vi "Create_Probe_Box.vi"(1 "Probe Volume":T1=[{"Max"=15.0, "Min"=-15.0}, {"Max"=250.0, "Min"=0.0}, {"Max"=15.0, "Min"=-15.0}] {"Min" format="%#.1f"; "Max" format="%#.1f"}, 2 "Probe Position":sgl[](array[numeric]) format="%.2f") -> (0 "Current Probe Volume":T1=[{"Max"=15.0, "Min"=-15.0}, {"Max"=250.0, "Min"=0.0}, {"Max"=15.0, "Min"=-15.0}] {"Min" format="%#.1f"; "Max" format="%#.1f"})   [LabVIEW 2014]
uses:
  Box_size.ctl
panel:
  # "(Relative to measurement position)"
  # "X                           Y                          Z"
  # "X                Y                  Z"
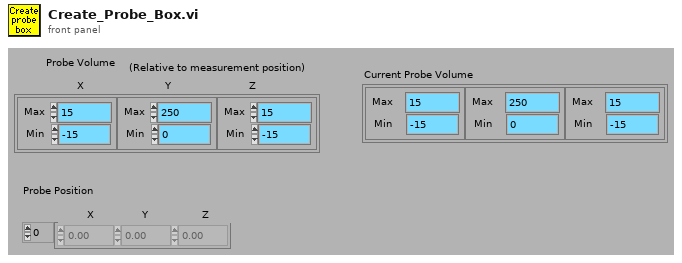
[diagram p1: front panel]
types:
  T1 = typedef "Box_size.ctl" = cluster{"Max":sgl, "Min":sgl}[]
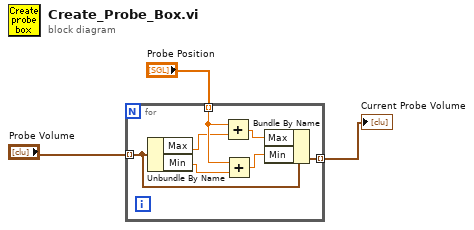
[diagram p0: block diagram]
diagram:
  n1 = for {
    tunnel: "Probe Volume" -> [w7] mode=indexing
    tunnel: "Probe Position" -> [w10] mode=indexing
    tunnel: [w4] -> w2 mode=indexing
    n2 = Unbundle By Name(w7) -> ("Max"=w9:sgl, "Min"=w8:sgl)
    n3 = Add(x=w10, y=w9) -> (x+y=w6:sgl)
    n4 = Add(x=w10, y=w8) -> (x+y=w5:sgl)
    n5 = Bundle By Name(cluster=w7, "Max"=w6, "Min"=w5) -> (w4:cluster{"Max":sgl, "Min":sgl})
  }
  "Current Probe Volume" <- w2
